vi "Write Command.vi"(8 "error in (no error)":errorcluster, 11 "command":string) -> (0 "error out":errorcluster, 2 "standard error":string, 3 "standard output":string)   [LabVIEW 2020, in "Manipulator CLI Driver.lvlib"]
uses:
  Manipulator CLI Driver.lvlib
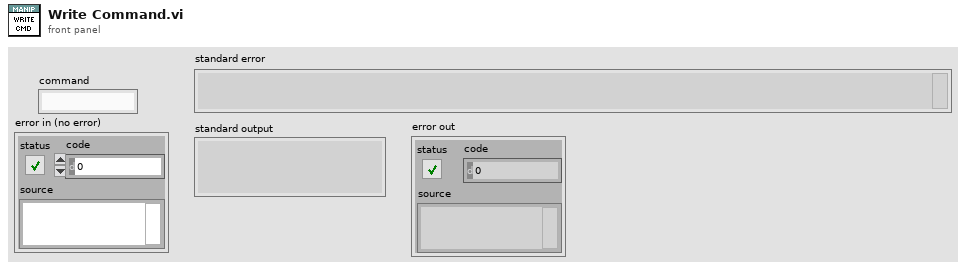
[diagram p1: front panel]
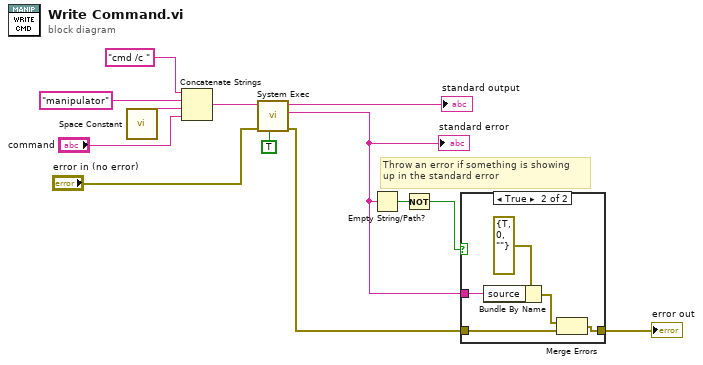
[diagram p0: block diagram]
diagram:
  # "Throw an error if something is showing\nup in the standard error"
  n1 = call <vilib>:"Space Constant.vi"() -> ("String"=w11:string)
  n2 = Concatenate Strings("cmd /c ", "manipulator", w11, "command") -> (w9:string)
  n3 = call <vilib>:"System Exec.vi"("run minimized? (F)"=TRUE, "error in (no error)"="error in (no error)", "command line"=w9) -> ("error out"=w5:errorcluster, "standard error"=w2:string, "standard output"=→"standard output":string)  [unwired: 5 in, 1 out]
  "standard error" <- w2
  n4 = Empty String/Path?(string/path=w2) -> (empty?=w6:bool)
  n5 = Not(x=w6) -> (.not. x?=w3:bool)
  n6 = case shown="True" w3 {
    tunnel: w5 -> [w14 w19]
    tunnel: [w14 w16] -> w4
    tunnel: w2 -> [_ w17]
    frame False {
    }
    frame True {
      n7 = Bundle By Name(cluster=errorcluster {"status"=TRUE, "code"=0, "source"=""} ("error in (no error)"), "source"=w17) -> (w15:errorcluster)
      n8 = Merge Errors(w15, w19) -> (w16:errorcluster)
    }
  }
  "error out" <- w4
